vi "TS DAC Acq Start.vi"(8 "error in (no error)":errorcluster, 11 "Generic Test Stand in":refnum<class "Generic Test Stand.lvclass">) -> (0 "error out":errorcluster, 3 "Generic Test Stand out":refnum<class "Generic Test Stand.lvclass">)   [LabVIEW 2019, in "Generic Test Stand.lvclass"]
uses:
  Generic Test Stand.lvclass
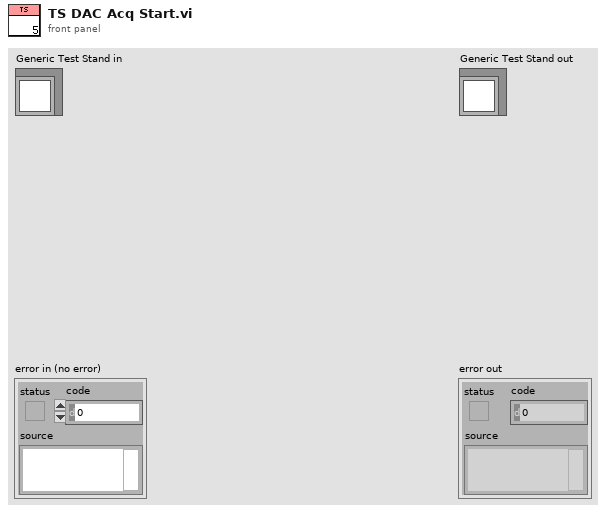
[diagram p1: front panel]
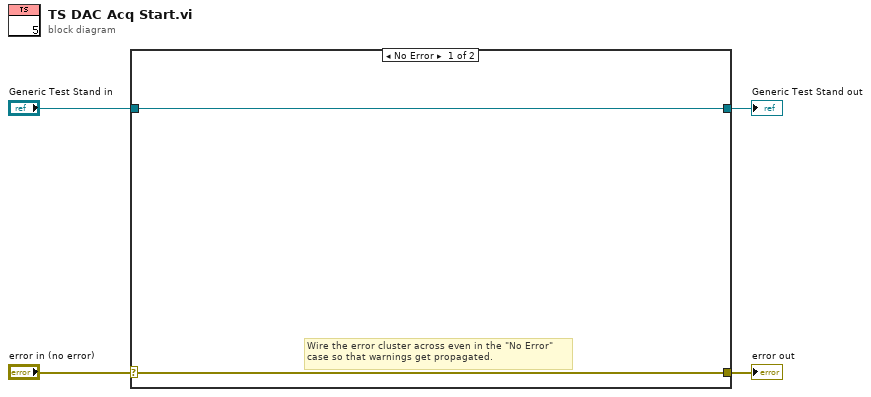
[diagram p0: block diagram]
diagram:
  n1 = case shown="No Error" "error in (no error)" {
    selector: "error in (no error)" -> [w5 w8]
    tunnel: [w5 w8] -> w3
    tunnel: [w6 w7] -> w1
    tunnel: "Generic Test Stand in" -> [w6 w7]
    frame No Error {
      # "Wire the error cluster across even in the \"No Error\"\ncase so that warnings get propagated."
    }
    frame Error {
    }
  }
  "error out" <- w3
  "Generic Test Stand out" <- w1
